vi "PCO_GetSegmentStruct.vi"(8 "error in (no error)":errorcluster {"code" format="%x"}, 10 "wSegment":u16, 11 "ph":u64) -> (0 "error out":errorcluster {"code" format="%x"}, 1 "strSegment":T1, 2 "ErrorMessage":i32 format="%x", 3 "ph out":u64)   [LabVIEW 2019, in "SDK.lvlib" / "ImageInformation.lvlib"]
doc: "<b>Description:</b>\nInformation about previously recorded images is queried from the camera and the variables of the PCO_Segment structure are filled with this information. These returned parameters depend on the camera settings, which have been active during the last recording to the dedicated segment.\nThe PCO_Segment structure includes also information about count of images in the segment and the last SoftROI settings, which are pure virtual and depend only on settings in the API.\n\n<b>Supported camera type:</b>\npco.dimax, pco.1200, pco1600, pco.2000, pco.4000\n\n<b>Descriptor dependency:</b>\ndwGeneralCapsDESC1: NO_RECORDER"
uses:
  ImageInformation.lvlib
  Structures/Structures.lvlib
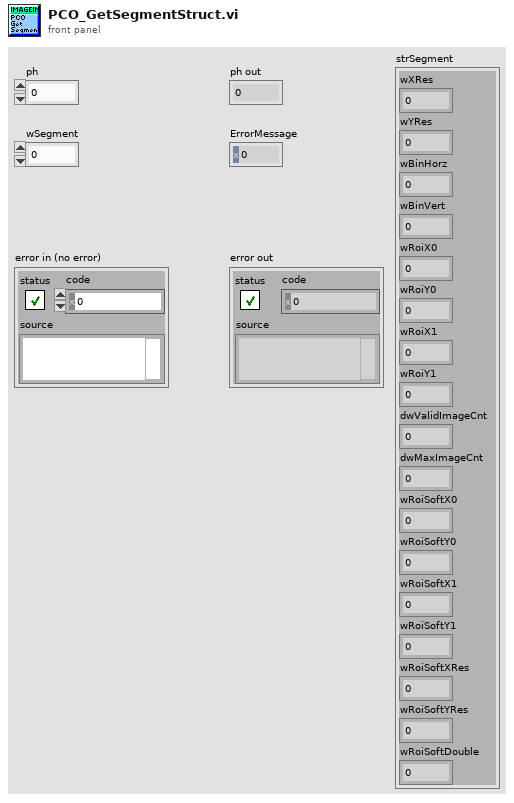
[diagram p1: front panel]
types:
  T1 = cluster{"wXRes":u16, "wYRes":u16, "wBinHorz":u16, "wBinVert":u16, "wRoiX0":u16, "wRoiY0":u16, "wRoiX1":u16, "wRoiY1":u16, "dwValidImageCnt":u32, "dwMaxImageCnt":u32, "wRoiSoftX0":u16, "wRoiSoftY0":u16, "wRoiSoftX1":u16, "wRoiSoftY1":u16, "wRoiSoftXRes":u16, "wRoiSoftYRes":u16, "wRoiSoftDouble":u16}
  T2 = cluster{"wSize":u16, "wXRes":u16, "wYRes":u16, "wBinHorz":u16, "wBinVert":u16, "wRoiX0":u16, "wRoiY0":u16, "wRoiX1":u16, "wRoiY1":u16, "ZZwAlignDummy1":u16, "dwValidImageCnt":u32, "dwMaxImageCnt":u32, "wRoiSoftX0":u16, "wRoiSoftY0":u16, "wRoiSoftX1":u16, "wRoiSoftY1":u16, "wRoiSoftXRes":u16, "wRoiSoftYRes":u16, "wRoiSoftDouble":u16, "ZZwDummy":cluster{u16, u16, u16, u16, u16, u16, u16, u16, u16, u16, u16, u16, u16, u16, u16, u16, u16, u16, u16, u16, u16, u16, u16, u16, u16, u16, u16, u16, u16, u16, u16, u16, u16}}
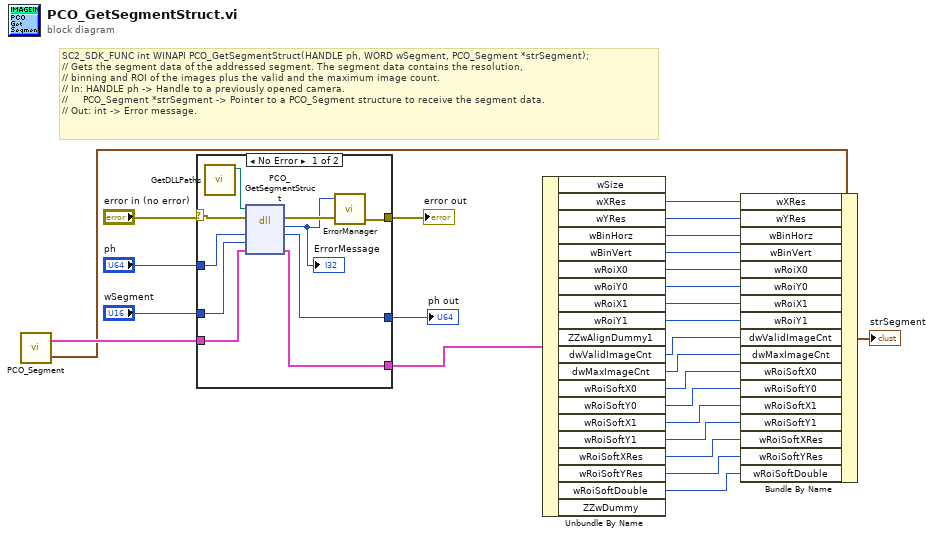
[diagram p0: block diagram]
diagram:
  # "SC2_SDK_FUNC int WINAPI PCO_GetSegmentStruct(HANDLE ph, WORD wSegment, PCO_Segment *strSegment);\n// Gets the segment data of the addressed segment. The segment data contains the resolution,\n// binning and ROI of the images plus the valid and the maximum image count.\n// In: HANDLE ph -> Handle to a previously opened camera.\n//     PCO_Segment *strSegment -> Pointer to a PCO_Segment structure to receive the segment data.\n// Out: int -> Error message."
  n1 = call "PCO_Segment.vi"() -> ("PCO_Segment"=w19:T1, "PCO_Segment_Raw"=w21:T2)  [unwired: 4 in, 2 out]
  n2 = case shown="No Error" "error in (no error)" {
    selector: "error in (no error)" -> [w31 w39]
    tunnel: "ph" -> [w36 w38]
    tunnel: [w35 w38] -> w25
    tunnel: "wSegment" -> [w34 _]
    tunnel: w21 -> [w33 w37]
    tunnel: [w32 w37] -> w20
    tunnel: [w29 w39] -> w23
    frame No Error {
      n3 = call "GetDLLPaths.vi"() -> ("SC2_Cam_Path"=w27:path)  [unwired: 9 in, 2 out]
      n4 = dll-call lib="?" fn="PCO_GetSegmentStruct"(path in=w27, error in=w31, "ph"=w36, "wSegment"=w34, "strSegment"=w33) -> (error out=w30:errorcluster, "return type"=w28:i32, "ph"=w35:u64, "strSegment"=w32:T2)  [unwired: 2 in, 1 out]
      "ErrorMessage" <- w28
      n5 = call "ErrorManager.vi"("error in (no error)"=w30, "error code"=w28) -> ("error out"=w29:errorcluster)  [unwired: 3 in]
    }
    frame Error {
    }
  }
  "ph out" <- w25
  "error out" <- w23
  n6 = Unbundle By Name(w20) -> ("wXRes"=w18:u16, "wYRes"=w17:u16, "wBinHorz"=w16:u16, "wBinVert"=w15:u16, "wRoiX0"=w14:u16, "wRoiY0"=w13:u16, "wRoiX1"=w12:u16, "wRoiY1"=w11:u16, "dwValidImageCnt"=w10:u32, "dwMaxImageCnt"=w9:u32, "wRoiSoftX0"=w8:u16, "wRoiSoftY0"=w7:u16, "wRoiSoftX1"=w6:u16, "wRoiSoftY1"=w5:u16, "wRoiSoftXRes"=w4:u16, "wRoiSoftYRes"=w3:u16, "wRoiSoftDouble"=w2:u16)  [unwired: 3 out]
  n7 = Bundle By Name(cluster=w19, "wXRes"=w18, "wYRes"=w17, "wBinHorz"=w16, "wBinVert"=w15, "wRoiX0"=w14, "wRoiY0"=w13, "wRoiX1"=w12, "wRoiY1"=w11, "dwValidImageCnt"=w10, "dwMaxImageCnt"=w9, "wRoiSoftX0"=w8, "wRoiSoftY0"=w7, "wRoiSoftX1"=w6, "wRoiSoftY1"=w5, "wRoiSoftXRes"=w4, "wRoiSoftYRes"=w3, "wRoiSoftDouble"=w2) -> (→"strSegment":T1)
